vi "MailWake.vi"() -> ()   [LabVIEW 2012]
uses:
  Config.ctl
panel:
  in  "Test":bool
  in  "Save":bool
  in  "配置信息":T1[](array[typedef])=[{"主题"="haobo.li", "Mac Address"="脯o'j\u000e"}]
  out "Mac Address":string
  out "message":string="There are no messages on the mail server."
  out "Messages:":string[][](table)
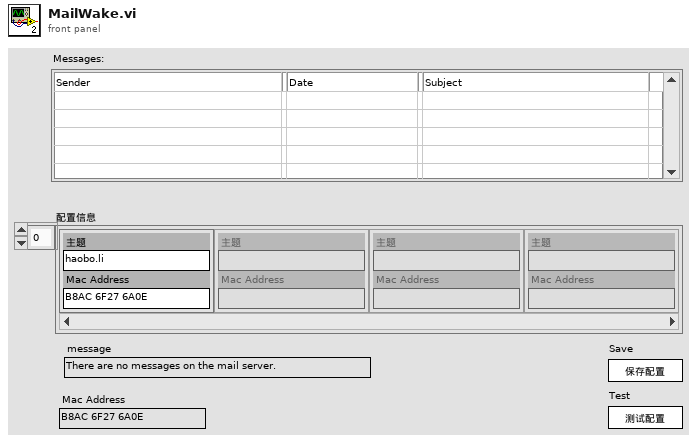
[diagram p1: front panel]
types:
  T1 = typedef "Config.ctl" = cluster{"主题":string, "Mac Address":string}
  T2 = enum32{"invalid app kind", "Development System", "Run Time System", "Student Edition", "Embedded LabVIEW", "Evaluation", "Custom"}
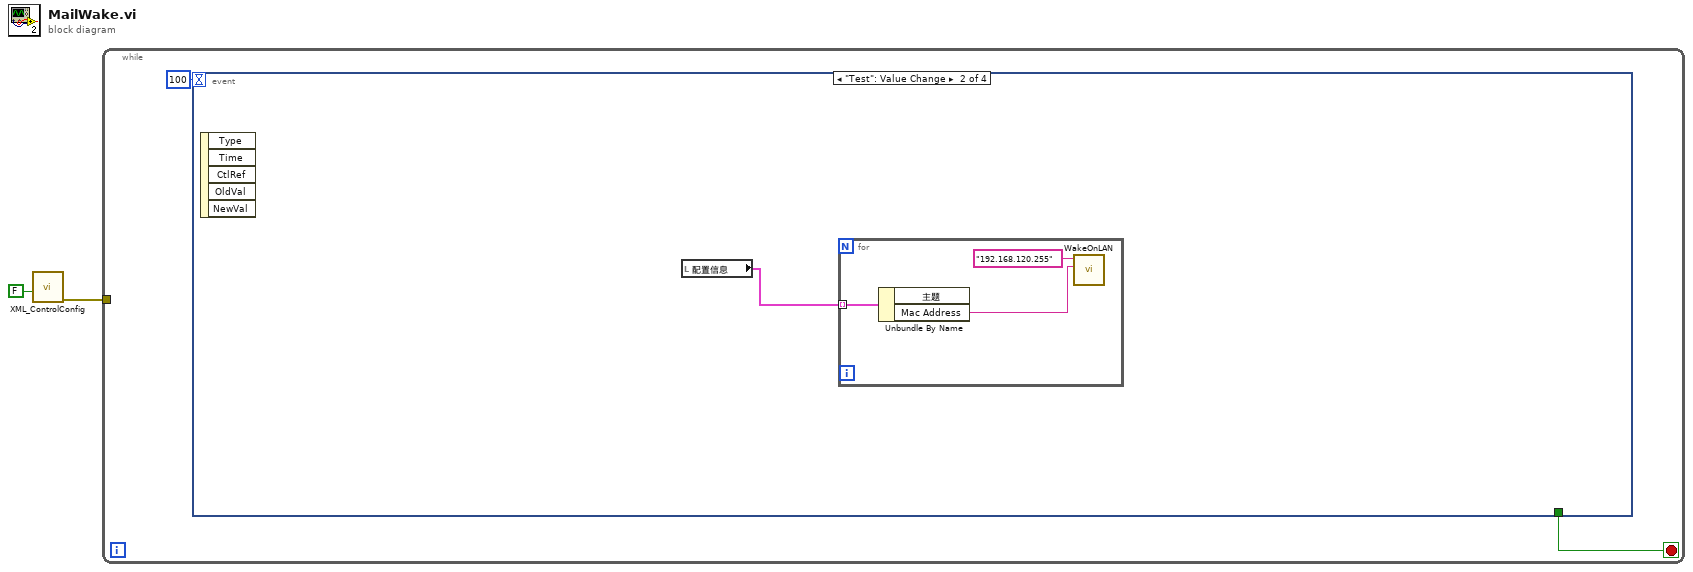
[diagram p0: block diagram]
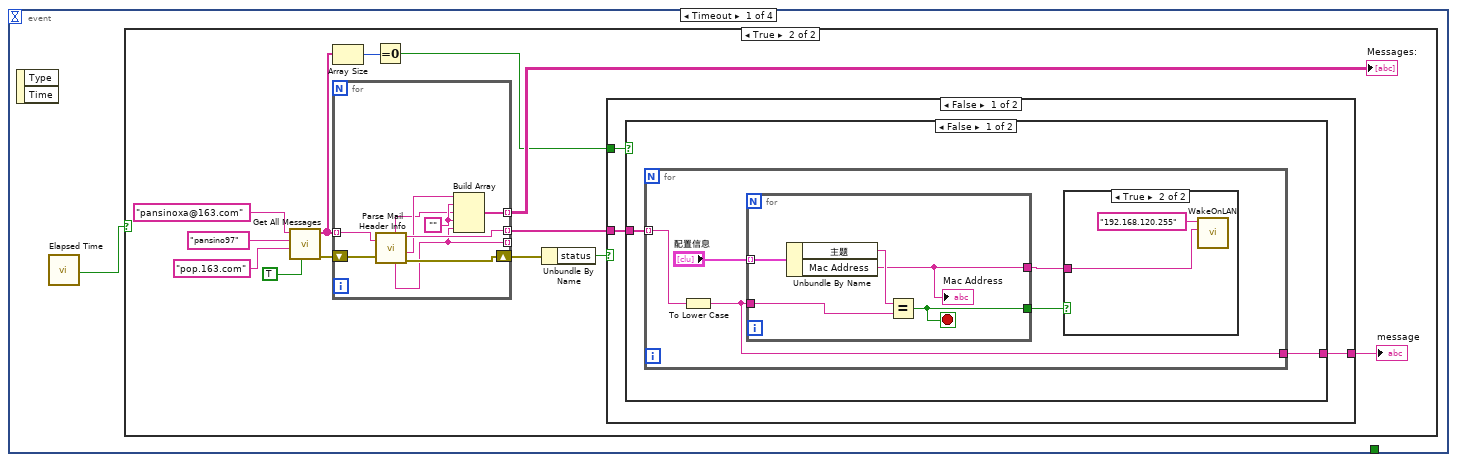
[diagram p2: hidden frame]
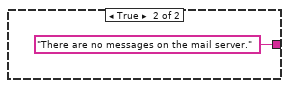
[diagram p5: hidden frame]
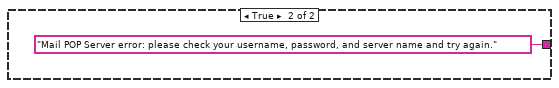
[diagram p6: hidden frame]
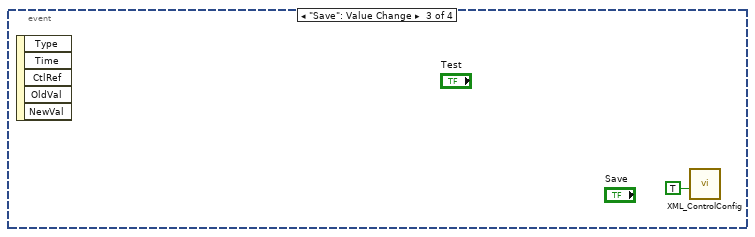
[diagram p7: hidden frame]
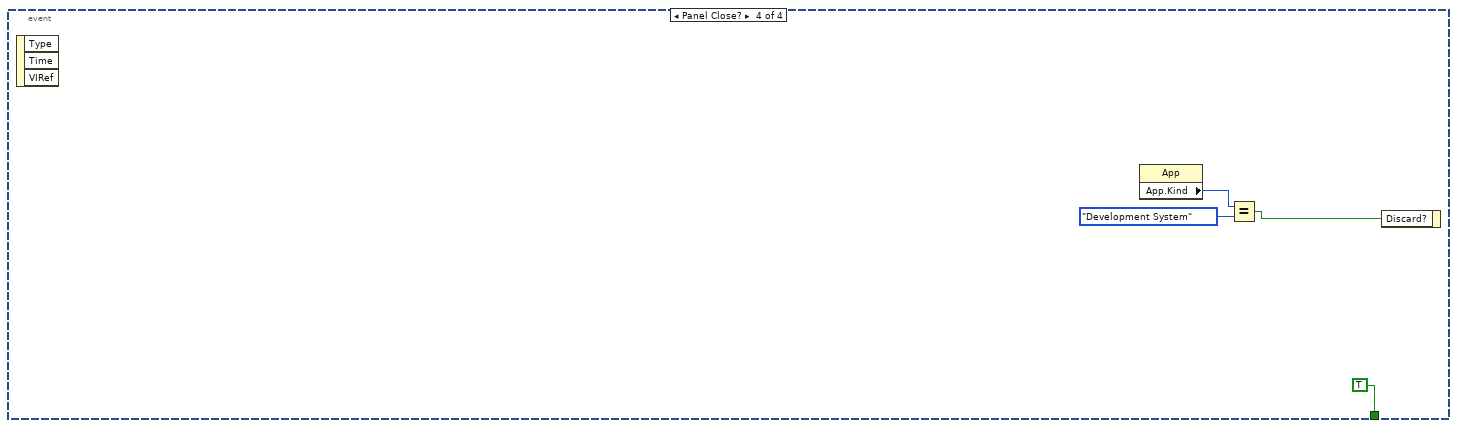
[diagram p8: hidden frame]
diagram:
  n1 = call "XML_ControlConfig.vi"("Save?"=FALSE) -> ("error out"=w2:errorcluster)  [unwired: 10 in]
  n2 = while {
    tunnel: w2 -> [_]
    stop <- w3 stop-if-true
    n3 = event shown="[1] \"Test\": Value Change" {
      selector: _ -> [_ _ _ _]
      dyn-events: _ -> [_ _ _ _]
      timeout: 100 -> [_ _ _ _]
      tunnel: [_ _ _ TRUE] -> w3
      event Timeout {
        n4 = event-data() -> ()  [unwired: 1 in, 2 out]
        n5 = call "Elapsed Time"() -> ("Time has Elapsed"=w5:bool)  [unwired: 12 in, 7 out]
        n6 = case shown="True" w5 {
          frame False {
          }
          frame True {
            n7 = call "Get All Messages.vi"("delete from server (Y)?"=TRUE, "POP server name/IP"="pop.163.com" ("POP server:"), "password"="pansino97" ("Password:"), "username"="pansinoxa@163.com" ("Username:")) -> ("error out"=w14:errorcluster, "message array"=w9:string[])  [unwired: 4 in, 1 out]
            n8 = Array Size(array=w9) -> (size(s)=w8:i32)
            n9 = for {
              tunnel: w9 -> [w46] mode=indexing
              shift-right: [w44] -> w12
              shift-left: w14 -> [w45]
              tunnel: [w43] -> w13 mode=indexing
              tunnel: [w41] -> w10 mode=indexing
              tunnel: [w38] -> _ mode=indexing
              w40 = ""
              n10 = call "Parse Mail Header Info.vi"("Message Content"=w46, "error in (no error)"=w45) -> ("Date"=w39:string, "Subject"=w38:string, "Message Content out"=w43:string, "From"=w42:string, "error out"=w44:errorcluster)  [unwired: 1 out]
              n11 = Build Array(w42, w40, w39, w40, w38) -> (w41:string[])
            }
            "Messages:" <- w10
            n12 = Equal To 0?(x=w8) -> (x = 0?=w7:bool)
            n13 = Unbundle By Name(w12) -> ("status"=w11:bool)
            n14 = case shown="False" w11 {
              tunnel: w13 -> [w21 _]
              tunnel: w7 -> [w20 _]
              tunnel: [w19 "Mail POP Server error: please check your username, password, and server name and try again." ("message")] -> w6
              frame False {
                n15 = case shown="False" w20 {
                  tunnel: w21 -> [w23 _]
                  tunnel: [w22 "There are no messages on the mail server." ("message")] -> w19
                  frame False {
                    n16 = for {
                      tunnel: w23 -> [w28] mode=indexing
                      tunnel: [w27] -> w22
                      n17 = To Lower Case(string=w28) -> (all lower case string=w27:string)
                      n18 = for {
                        tunnel: [w34] -> w26
                        tunnel: w27 -> [w35]
                        tunnel: [w31] -> w24
                        tunnel: "配置信息" -> [w33] mode=indexing
                        stop <- w34 stop-if-true
                        n19 = Unbundle By Name(w33) -> ("主题"=w32:string, "Mac Address"=w31:string)
                        "Mac Address" <- w31
                        n20 = Equal?(x=w32, y=w35) -> (x = y?=w34:bool)
                      }
                      n21 = case shown="True" w26 {
                        tunnel: w24 -> [_ w29]
                        frame False {
                        }
                        frame True {
                          n22 = call "WakeOnLAN.vi"("Mac Address"=w29, "IP of the computer to control"="192.168.120.255") -> ()  [unwired: 10 in]
                        }
                      }
                    }
                  }
                  frame True {
                  }
                }
              }
              frame True {
              }
            }
            "message" <- w6
          }
        }
      }
      event "Test": Value Change {
        n23 = event-data() -> ()  [unwired: 1 in, 5 out]
        n24 = local read "配置信息"() -> (w47:T1[])
        n25 = for {
          tunnel: w47 -> [w50] mode=indexing
          n26 = Unbundle By Name(w50) -> ("Mac Address"=w48:string)  [unwired: 1 out]
          n27 = call "WakeOnLAN.vi"("Mac Address"=w48, "IP of the computer to control"="192.168.120.255") -> ()  [unwired: 10 in]
        }
      }
      event "Save": Value Change {
        n28 = event-data() -> ()  [unwired: 1 in, 5 out]
        n29 = call "XML_ControlConfig.vi"("Save?"=TRUE) -> ()  [unwired: 10 in, 1 out]
      }
      event Panel Close? {
        n30 = event-data() -> ()  [unwired: 1 in, 3 out]
        n31 = property class="App"() -> ("App.Kind"=w54:T2)  [unwired: 2 in, 2 out]
        n32 = Equal?(x=w54, y=T2."Development System") -> (x = y?=w52:bool)
        n33 = event-data("Discard?"=w52) -> ()  [unwired: 1 in, 1 out]
      }
    }
  }
